vi "BasicGrid.vi"() -> ()   [LabVIEW 2015]
panel:
  out "Map":u16[][](array[ring])
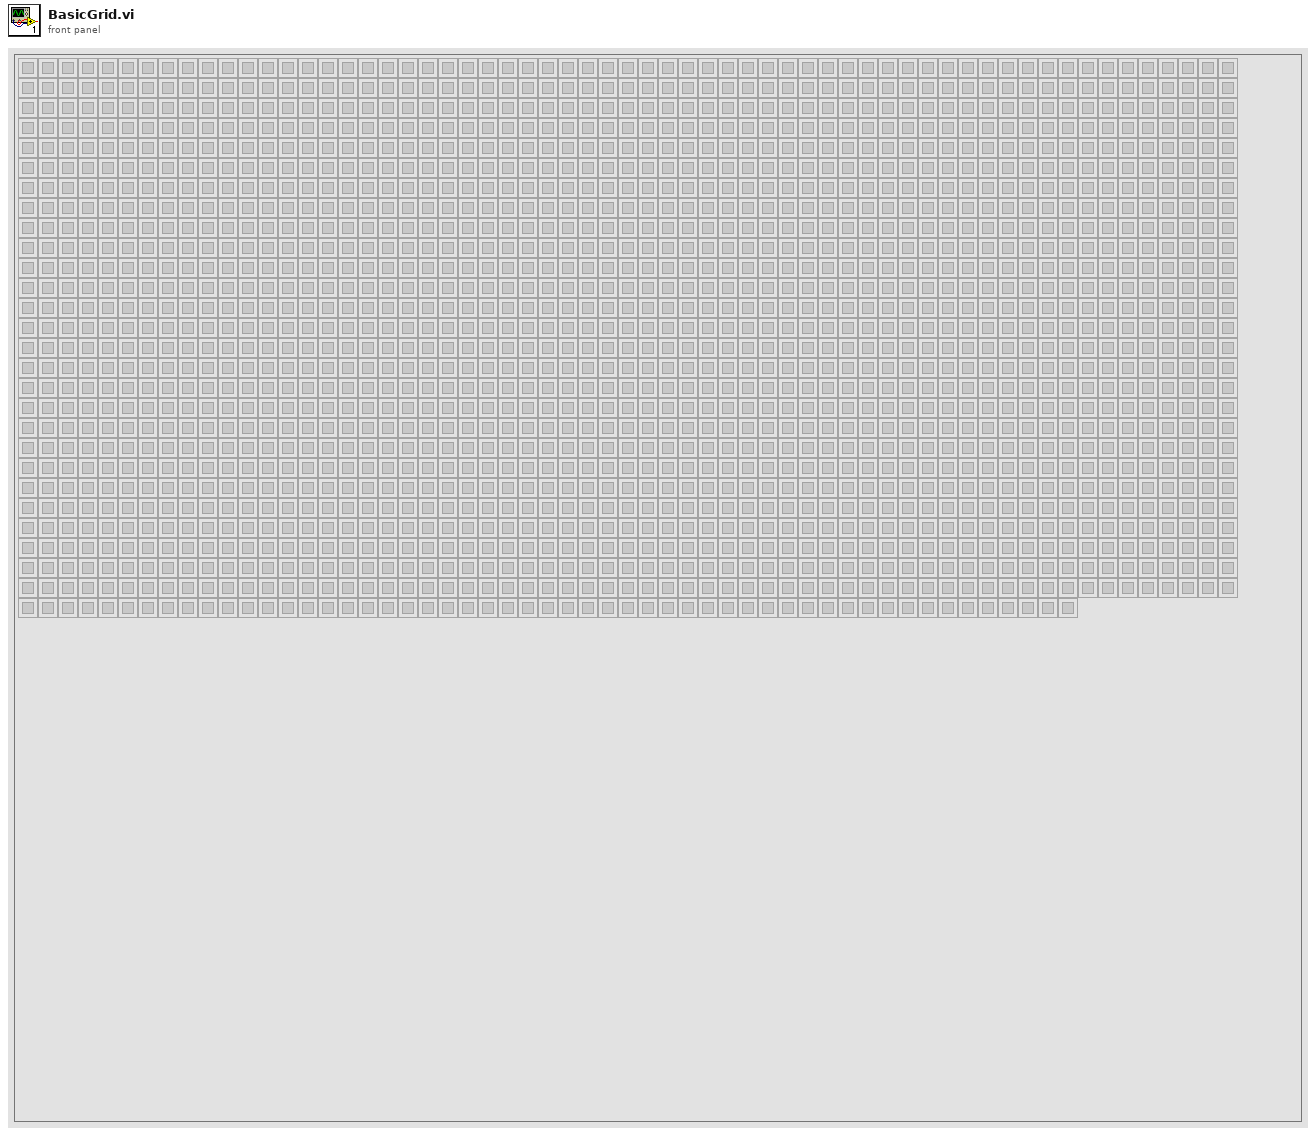
[diagram p1: front panel]
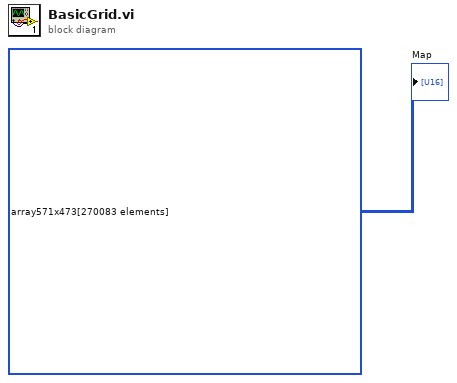
[diagram p0: block diagram]
diagram:
  "Map" <- i32[][] array571x473[270083 elements]
